vi "Supplementary Fig.9.vi"() -> ()   [LabVIEW 2018]
uses:
  cd616403-dbdb-4a2d-b889-8bc5e4dbac0b.vi
  <vilib>/Analysis/baseanly.llb/Mean (DBL).vi
  <vilib>/Array/Sort 2D Array - Pop Stack.vi
  <vilib>/Array/Sort 2D Array - Push Stack.vi
  <vilib>/Utility/file.llb/Read Delimited Spreadsheet (string).vi
  <vilib>/Utility/file.llb/Write Delimited Spreadsheet (string).vi
  <vilib>/Analysis/NI_AALBase.lvlib
  <vilib>/Analysis/NI_AALPro.lvlib
  <vilib>/gmath/NI_Gmath.lvlib
panel:
  out "appended path":path
  out "coerced(x)":dbl[](array[numeric])=[1.7871616862624315, 4.7491649613370654, 3.3004814514035252, 1.8375936522629628, 3.202316398326516, 4.319522827090855, 3.6552232003410356, 4.668576210850217, 5.083284828825093, 6.10710953942415, 1.646654574018751, 3.7290215132163573, 6.098038325809161, 5.656422627696404, 1.7758128410410414, 3.761570516262, 4.165469016958864, 3.753437357839156, 1.8892827388338778, 4.736459568723037, 1.9574851838284406, 1.920321934057286, 1.925685182031331, 3.788311995806621, 3.0656954505481155, 3.3434841534854978, 3.244966710765227, 1.94311088130418, 3.262816320637847, 1.5462436499858399, 4.548235957251834, 3.6315283681364328, 5.664268399574894, 3.7876699725560314, 1.5612286705468439, 3.287096907045537, 1.6510086873136212, 3.624242770804696, 5.724032802363539, 4.606639647843998, 5.72864322441162, 4.593664726193712, 3.681475732616018, 1.9120549299762257, 6.051355605980825, 4.229281804790069, 3.3406395414558507, 1.8857089065912496, 5.028477399370969, 1.8779605152106047, 1.9111177530654646, 4.664931537320069, 4.186588228645763, 3.2553177687757553, 5.145740103560326, 1.8655992677296291, 1.8046874224504181, 3.0833404640629962, 5.114735680413688, 1.671303972442136, 6.15886900181359, 1.6937395643797195, 3.2536286190286905, 1.842378459360618, 3.7411416491379326, 3.687868246017935, 4.6687925790572375, 1.7586356265470842, 1.8767109641028685, 6.223402134828333, 1.9218572626605044, 3.262014311657234, 1.858320784403082, 4.229963891029505, 1.7347160978595189, 1.685903113936927, 3.700740882251585, 1.7486080037864187, 1.3279294574595724, 3.27544870212411, 3.1368795583033524, 5.616373614885827, 4.268739670631767, 4.253677140988713, 3.6598944224590073, 1.6651274746829139, 4.567994774469708, 1.8542816659595915, 1.688649332258707, 3.29103595985378, 1.8177153438196487, 6.156642024225981, 5.693990388178911, 3.7467283566933944, 1.8453752547517892, 1.917568921369865, 3.2166573059812857, -6.0, 3.89516119392203, 4.232066120234996, 4.139995221043025, 4.973110775936315, 5.608411862084524, 6.134742821848983, 3.291437641822879, 1.8493786914051453, 6.155209143744587, 1.9469302220382134, 3.15342082229652, 1.9749257606375414, 3.343048402338881, 4.2227229180842905, 1.747201555363561, 1.9147522538662338, 1.8587717675188418, 5.662609144117798, 1.9579770221178325, 1.9867431460029874, 3.7904353802213953, 4.230297805342971, 3.2424672304005973, 1.7245832822394196, 5.085249166237611, 1.6080931386501884, 1.613418966188712, 5.140685993693935, -6.0, 1.8719017949112369, 4.2036571121076935, 4.613226980723122, 3.715812337259548, -6.0, 6.061258340225863, 3.7784475546863354, 3.175380674901726, -6.0, 4.615776455361565, 5.184458666423934, 2.025873248470572, 1.73105429451897, 1.716152423032959, 2.036713590493777, 1.574951505953829, 1.8586171256624935, 3.8601284514654104, 4.257991110958849, 1.2065423321612012, 5.611842616698198, 4.579328211355799, 4.111465632573334, 5.146009633606169, 4.567990817904687, 1.9354997588134508, 0.231812761540904, 1.8926221225819462, 3.220052434083975, 3.1463031104018313, 3.22934925835474, 3.327581039341003, 4.345931379092285, 2.0190197998590023, 1.8508399889779195, 1.8366049172096368, 3.1947954331244874, 4.158453183730934, 4.590854029283031, 1.5620256852329995, 1.9893632927815357, 1.659705825153652, 3.795380915100212, 1.195897550086908, 6.0964899066291665, 4.293081716415471, 4.187708236455775, 1.8949490451589543, 5.297148552742282, 3.5382709525514318, 3.578648565876757, 3.277535694974436, 1.707088847431416, 3.7419078216422346, 1.8807526839232078, 6.117955417135745, 3.7912239842840867, 3.6896107042372273, 1.6523256191092637, 1.7960841364158975, 1.636221470769201, 5.155760366117264, 5.656387939814442, 1.3357976408128798, 4.348441122733338, 3.879302402815981, 1.7524323251076086, 3.325504807507367, 1.9436913184974423, 3.773197277176825, 1.6851970426101552, 3.357871833347651, 1.5597183420965208, 3.3109889271775175, 3.7365065137012836, 4.6334044609059575, 1.8003185815047131, 1.7383792054463407, 1.6498374438002832, 3.7494393752685258, 1.460031997854308, 1.7920524290693296, 1.8162541496139923, 0.3871565974248339, 4.612645757412732, 4.6592514227918125, 4.564963074244081, 0.9429870149856682, 1.7270964549130992, 6.048468648027366, 5.04871188235065, 4.240467531757491, 3.270178269411716, 5.0804248855576155, 5.820448008477603, 3.768068761017986, 6.1524394738365356, 4.1177625818053185, 6.111113088204756, 1.5366038643690156, 1.6606280398831155, 3.7487600956387754, 4.757735202780968, 1.945793554112217, 3.807325140809996, 1.8712704526987887, 3.735923451922705, -6.0, 5.115000993235436, 4.380398873391102, 1.953798786138667, 4.636272145582572, 1.8273375076454474, 1.5459102430749714, 6.0846786930998915, 3.0890760065506027, 1.5470917850623196, 3.414232163593886, 1.8784324342398588, 5.568704779949148, 1.7588686726502683, 3.2913100959369586, 3.7322491342602486, 5.661382491336868, 1.4119982524594679, 1.9465745331390063, 1.7300309182128206, 4.696356057813045, 4.964053988335164, 4.695631209986867, 5.6621629936392734, 5.6265410460358325, 4.134527945665677, 4.138785260823419, 4.674190604292248, 1.930554942741988, 5.774946746787386, 4.307050909108307, 3.257989350115037, 1.3904335782414181, 3.6408565707327174, 3.262074232050821, 3.2764631759901555, 1.848577584401121, 1.827328433234382, 1.8960337747362794, 3.3041030370948374, 4.659246088467658, 3.210503304520497, 6.133408069554185, 3.5826212864175275, 6.111857614641569, 1.696478917640413, 3.6241546068461754, 5.22798044456426, 3.7519995544236524, 3.1219975683106997, 5.615946903414847, 3.6701121258372478, 4.697000602278537, 4.753643931101217, 5.656789429450875, 1.808528506417126, 4.7160234241873855, 3.5683886756500516, 5.639204986940518, 4.612624965415669, -6.0, 3.787560696986183, 5.10881077367408, 3.3537508122386126, 1.7718675509127513, 3.729390780351592, 1.1802873430259595, 3.0444549741493296, 4.24672540031586, 5.146264484882083, 3.28179514705405, 4.71404906709892, 5.109900283765078, 3.6140930051711266, 1.946678471551835, 3.6605074662327364, 1.8327673878842443, 3.242524603781917, 5.644941262625613, 1.8207855178820165, 4.7124578651337865, 1.8310254890264943, 1.7233969931626747, 6.084744741056078, 3.7447894548142115, 4.591053763793992, 5.690718937826536, 4.621081782709175, 1.6154774441434179, -6.0, 1.738930340473572, 4.2861274968388114, 4.186865946356676, 5.089454194286781, 1.4444445377463588, 3.2266824238862917, 1.8541422971015722, 6.144774691882833, 6.081983773027188, 5.665405834035932, 3.230297633583582, 1.9813658717460187, 4.268715548550998, 3.1603284853374203, 3.1925795297887505, 4.775281033677114, 4.241797375586176, 4.176880540064573, 1.9201767641917182, 6.085705663824028, 5.7079581669094015, 1.5413908216067886, 5.636004373210665, 5.0663995272902556, 4.76324257120765, 3.788440571838505, 3.220202113342905, 1.4773250647190024, 1.4502453967797377, 1.7988832448499659, 5.6146213167944, 5.075176622438101, 1.6190472574726358, 6.039643381801598, 2.003610467075469, 5.0517553831061734, 0.492511191708194, 6.166115565545919, 3.2517453701832015, 3.2807633335959205, 3.7531912971441037, 1.866488852235544, 1.815261860210051, 1.7154256234981156, 1.8487750622102372, 6.135926272641424, 3.1570698301320657, 1.8960117589378596, 0.3204447869350835, 1.443174883256306, 2.0360349109813636, 5.28182732836023, 5.077250657859839, 0.8087337027630944, 1.8396089759074978, 3.6395594044778523, 1.7408184121349726, 1.793196426632025, 1.893985596206091, 1.7838410092168282, 1.7558360874452674, 3.722918798068077, 4.216885293889205, 5.050524628381662, 5.460371696735989, 5.133147292731508, 3.7043513164181427, 6.087569430540786, 5.162414361098457, 1.930402193876784, 1.8487806604029207, 4.005641262803538, 1.4332832475963648, 3.0590477068872386, 1.8461360713964619, 4.5099930962861565, 1.769126455955212, 5.033360060420678, 1.8190000624294527, 3.255128164822189, 4.212433313348358, -6.0, 3.316188486924122, 3.23019364138835, 3.7957278405824186, 1.4168099822318794, 5.1176017436748795, 4.2556053094661435, 5.093984562350116, 6.052213040115122, 3.1797507208319966, 1.4397455668401162, 1.6665840182464593, 6.153468876985319, 3.7308976534322444, 3.2906244569156007, 3.1549827650297084, 5.5880803202832965, 5.200358521823363, 1.928687791543826, 1.0120576203426224, 3.7468547587589343, 2.014619310619202, 4.664894471832111, 4.154782912356386, 6.116253447268662, 1.7906457672949294, 5.142509396818882, 1.9302839395891997, 4.191792649357379, 6.1438367723348355, 5.107781301970035, 3.6752721725438486, 1.925946883606187, 3.644826317829624, 3.7219899568797676, 3.9084807388586325, 3.2068581232230047, 5.147884754186237, -6.0, -6.0, 5.155258937957506, 4.555483154870481, 4.564905256987634, 1.8124903349442976, 3.154384497999989, 1.7868050385923993, 1.9289894925706583, 4.682905174953122, 6.0099354084690395, 3.3482319844618527, 1.611920203703713, 4.2221213418770445, 4.631661772685009, 1.674581881337848, 3.153515741834732, -6.0, 1.8620458303853011, 5.133997735463562, 1.7070586592824344, 1.8156932061674182, 5.08617481260544, 3.229187606888848, 5.605858992814849, 3.341251367424632, 3.1100966149814386, 5.173982465505348, 1.7834843399537785, 4.176725530975806, -6.0, 1.3606300071078101, 5.614879505481419, 1.8472931155004508, 1.6675136471397716, 3.7647186386378393, 6.123919597813203, 5.612762159529842, 5.690864478125958, 4.226246546698345, 4.255129044053117, 4.224462485105966, 4.694285966418743, 1.7184351611506758, 4.308963598546429, 5.207854509662446, 3.259713201981584, 6.067584503363792, 1.9358964298642602, 4.5663698129989685, 5.559759910512286, 0.3772699976247565, 1.5849254956703018, 1.8099162418539883, 1.9057342223596525, 4.249212707075614, 3.659011694892542, 3.828125478045003, 5.148714404505429, 1.6937199772983755, 6.1305664927082235, 3.753363635354085, 1.8560809944746686, 1.8237788327232272, 1.7476136341099398, 1.9469056547501533, 1.7359181963061763, 3.7685500874730895, 4.612252527392213, 4.169260089075253, 1.6984437289208514, 5.137668501206944, 6.175225181467641, 5.110387621125306, 1.8012932081510782, 1.9170369382742187, 5.173343923381356, 1.6826841787193263, 4.646369542823793, 1.351420947529353, 5.072565356937414, 4.636950999500978, 3.1980169070011675, 1.841894549443889, 5.613278542057316, 1.870856108632458, 1.8811518844658337, 4.642382572974339, 4.574130441897333, 4.6276378076739215, 1.7349303542550565, 5.643352548525211, 3.315670571904706, 1.9605846447982938, 1.7467596358881765, 5.66461413145304, 4.6222431211728585, 4.697659831456345, 1.8597948948572858, 1.2922309214325127, 1.7973128311583562, 5.197177515139583, 5.139577946016122, 5.559318112318645, 1.5024674337519917, 1.7882296419507517, 1.8937981791462262, 4.216665846443737, 4.2049155018749325, 1.2999868932404879, 5.6636902441990875, 3.623030837766795, 3.6766757724641934, 1.5463202033208765, 5.594672564548696, 4.584906066216061, 1.8177443056467912, 1.8551448045518424, 5.642146794473806, 6.15704584106524, 5.650061703435735, 1.1366745358420236, 1.7348907339855077, 3.239356802215263, 1.659981016297658, 1.911891957674333, 5.668550823116212, 5.629572064716126, 5.622544246941823, 6.069322625000074, 3.7102615718886334, 3.1947643045065566, 1.850506717877915, 1.6400817618242793, 5.616024581303818, 1.8316798648455752, 3.318149857639774, 4.26915057172803, 3.693866079422621, 4.179602616586774, 1.7390011604991262, 3.225697530259093, 5.172738614517008, 1.5538744619810934, 3.310744051114857, 3.1686978379815773, 5.129756353458132, 5.70476630271836, 1.7211822468428042, 1.9540532026511654, 3.194357935517832, 3.3174144305947633, 1.9072173522866998, 3.75776587224984, 3.7493526929067933, 5.222013565096699, 4.164303207138102, 5.7397589855477325, 2.0198487241604077, 1.9508862448238076, 1.6488558482717486, 4.27562249979253, 5.669195781941759, 1.9690362793431593, 1.6687988685535902, 4.213065885194019, 1.8584040737295702, 4.654007941777578, 5.691763726913073, 4.736417113100859, 4.676010206847196, 6.071069665582147, 3.7601223339637757, 2.9427278237260164, 1.5312673257734735, 3.2341101643885217, -6.0, 5.707977662889405, 1.9532398118360457, 3.77732645744637, 6.085473348755801, 4.573065587919313, 5.039167075168178, 1.6395538694122245, 5.199620927314441, 1.9150225370062077, 5.662903033924214, 6.086457213036949, 3.3249809624804576, 6.0907846033375215, 3.686328732719376, 1.8096740907194235, 5.598084589983934, 5.153869461545504, 1.9018585596948745, 6.024745716223153, 3.7388530519535834, 1.8746099127797977, 3.069738947349552, 3.758685303480345, 1.7405609825601227, 1.7916819139301732, 2.0682621943565, 1.3596953476098517, 3.801460349644706, 1.8314904420799925, 4.559630609194131, 1.6371015529931428, 4.282149565236064, 3.310959824077987, 4.195632545872944, 3.675388300971693, -6.0, 1.5906428582687027, 5.11076516554976, 3.7338982130897596, 1.739339859535754, 1.9929178807168113, 4.303698457069036, 2.0571649996106194, 4.585681733692552, 3.170164635620533, 1.7444228138520603, 1.9570221804532706, 3.6330383834802196, 3.0712707495155542, 6.104329301798968, 5.110317753811609, 4.282847216418624, 5.670448898132594, 6.149655622163449, 4.593369687158319, 1.510252245324168, 1.7070337893551168, 6.1794066178585645, 1.9956145848613012, 6.0578482755461245, 1.852505501588917, 1.8816482180705145, 6.122879096743778, 1.8346215200335005, 3.2436629994988806, -6.0, 4.192278317351751, 3.2344836319791805, 5.560414501175136, 3.1580028991364926, 1.4085748705902077, 4.2021580092939335, 1.78492288846994, 5.75643114027947, 5.61315456730992, 4.241359051751067, 1.7302088626682521, 1.7218503591678622, 1.883122922564173, 5.643867938880513, 5.210922298309477, 6.072090858700979, 3.3545810131395597, 2.885467323080707, 1.4509108567828515, 1.8736304159176482, 6.076137642531447, 6.137882430759044, 3.2789705623310352, 3.887542932852534, 4.253875746851094, 5.046944625673959, 4.177095937722964, 3.5935793899248356, 1.8016059494695167, 4.250330767438225, 1.437692800983291, 3.72174761890751, 1.9293441848670025, 1.9625802085567017, 1.8721110746230343, 1.9249886744536406, 5.174540869140381, 2.006012042176779, 5.13007539577978, 3.2870833931380727, 1.7818630519774816, 6.205040767643756, 5.105176297628068, 1.6373887593191512, 1.8841608873885956, 0.6705110814541204, 4.662993957636156, 1.4703832768840923, 1.6214092525529635, -6.0, 1.923572672787042, 3.1585131875457373, 3.159249675294813, 3.0540390930783246, 1.1792309783974484, 1.7702569372194743, 3.1351053332356114, 1.9346549306612852, 5.693316291432743, 1.849038947737195, 4.670902458855315, 1.810986802204557, 3.717197118117848, 1.9288065118869488, 3.135066822934636, 1.7198271852013551, 3.766361179281768, 1.7607176128909743, 1.7675972857561029, 1.6868408845616951, 1.784344906730868, 5.59249605929259, 4.641124963216757, 3.686394071664694, 1.8554512138555737, 0.8980543038322548, 3.6350166843770815, 6.102073016901307, 5.670567120812509, 3.6763775562036214, 4.150032234643051, 3.7189935835093366, 3.6866891912543065, 3.4000710703278862, 4.148166318585837, 3.801241472238251, 2.970317740788838, 3.110029085492094, 5.039596460337458, 1.5257935719743616, 6.037572548800155, 3.1167185347135895, 1.8153753225836933, 3.650896403412224, 6.210434884080771, 1.9733572067777208, 6.072734490876358, 5.602695558881499, 0.19812543810824154, 3.5946428480086006, 1.8491402330568831, 4.256581366944582, 6.16299297762625, 3.3177528692463136, 1.8405877309890397, 3.315438376831165, 4.5960155758944, 3.762325605952752, 5.708177595302542, 1.7980308124089122, 4.580172802552053, 4.641906390261374, 5.10610802386794, 1.0689405810335257, 3.756412442700031, 1.6621445716194032, 3.2121212018296186, 1.0905656544893276, 6.109087292438708, 1.7045613830130464, 3.261673161737872, 5.181790291715928, 3.1526217948720956, 1.724238477694529, 5.0516087454053284, 5.60443081840953, 1.891660787597332, 4.628656650854219, 5.167457487372806, 3.7224958534254124, 1.7534798346663736, 3.659894063316376, 5.0922136390437895, 6.143659129937368, 3.7979943254692903, 3.6609603147185115, 1.7469422830568997, 1.7779425434591767, 1.842346443153822, 2.9176004909743227, 6.0771099380718665, 3.8080533872974343, 1.8403395465713333, 1.882529626513101, 1.9907894390633594, 3.1778268390962388, 1.4836044116851346, 3.2347671420248276, 5.047228208512596, -6.0, 3.647858983377213, 1.7092281666032834, 3.277446898096687, 4.764139205803011, 4.220692990286239, 1.937340090770517, 1.8172272616869425, 3.2984281834044937, 1.964154236159909, 1.6877948339082205, 1.721955712903482, 3.147619608788074, 1.8882588676054721, 5.061861465154706, 3.2620324502712643, 1.6535012043312718, 3.7628773180024275, 4.23113043665259, 1.9909072441489264, 1.6480611233110156, 1.568048214922474, 1.9572428199946788, 3.2650535117915815, 1.7491836605066104, 6.064137802913037, -6.0, 3.2375882284288355, 1.5697470552234873, 3.8452072239900326, -6.0, 3.2053157291452625, 5.572436608146442, 1.7583876308208932, 3.2203484445867243, 3.6855622073215066, 1.7137338646345357, 1.8145781931110154, 4.659981336525294, 5.102621410719233, 3.467056992374644, 5.674776916296293, 4.793654377310735, 5.640413965591396, 2.005531196709391, 1.8554325788835098, 3.242106531535169, 1.8098521622977441, 5.6989554698277765, 4.664518804707001, 3.2844750262388596, 5.628831986318144, 5.562795248124345, 6.065481335243661, 3.6801115696274476, 5.20422170449058, 3.856715864977252, 5.643818261701583, 1.847629847764977, 5.112968981436306, 6.08465903943604, 1.8369373419325807, 4.668592928087283, 1.8880375974637427, 3.0531999232556237, 3.6489968506814687, 1.7570638791239357, 1.8487613063445654, 1.8504654967727336, 5.642404851857281, 3.787394442355481, 0.7338503027874327, 3.6946134241299573, 4.175183268067918, 1.853993158131384, 4.728520025961949, 1.7998641995834261, 3.064062965934454, 4.8242654572654855, 1.840000263076598]
  in  "6peak boundary PE":dbl[](array[numeric])=[3.3500000000000036, 3.9500000000000024, 4.400000000000004, 5.0, 5.350000000000005, 7.0000000000000036] format="%_3g"
  in  "8peak boundary PE":dbl[](array[numeric])=[2.1999999999999997, 3.0999999999999996, 3.5999999999999996, 4.100000000000001, 4.450000000000001, 5.000000000000002, 5.350000000000002, 7.0] format="%_3g"
  in  "filename appendix":string
  in  "6peak(T)/8peak(F)":bool
  in  "8peak boundary FL":dbl[](array[numeric])=[2.8000000000000003, 3.5, 4.0, 4.4, 4.85, 5.35, 5.8500000000000005, 7.0] format="%_3g"
  in  "8peak-PE":dbl[](array[numeric])=[487.0, 1474.0, 4516.0, 11260.0, 34341.0, 107608.0, 260461.0]
  in  "8peak-FL":dbl[](array[numeric])=[771.0, 2106.0, 6262.0, 15183.0, 45292.0, 136258.0, 291042.0]
  in  "frame":i32=13
  in  "all":bool
  in  "channel":i32
  in  "file path":path
  in  "length(y) for bg calc":i32=24
  in  "length(x) for bg calc":i32=30
  out "loop index for stat analysis":i32=66
  out "loop index":i32=2999
  in  "load file":bool
  in  "save extracted data":bool
  out "size(s)":i32[](array[numeric])=[915, 7]
  in  "gating":bool=TRUE
  in  "index":i32=2
  in  "gating":T1(array[cluster])=[{"limit"=FALSE, "low"=0.0, "up"=500.0, "feature"=0}, {"limit"=TRUE, "low"=0.0, "up"=180.0, "feature"=1}, {"limit"=FALSE, "low"=0.0, "up"=1000000000.0, "feature"=2}, {"limit"=FALSE, "low"=0.30000000000000016, "up"=2.0, "feature"=3}, {"limit"=FALSE, "low"=0.0, "up"=1000000000.0, "feature"=4}, {"limit"=FALSE, "low"=27.0, "up"=60.0, "feature"=5}, {"limit"=FALSE, "low"=20.0, "up"=60.0, "feature"=6}] {"feature" items=["flow position", "seg area", "encircled intensity", "ratio", "total intensity", "peak x pos", "peak y pos"]}
  in  "feature names":string[](array[string])=["flow position", "seg area", "encircled intensity", "ratio", "total intensity", "peak x pos", "peak y pos"]
  in  "aperture diameter":dbl=10.0
  in  "Threshold Limits":cluster{"Lower value":sgl, "Upper value":sgl}={"Lower value"=0.29999992, "Upper value"=65000.0} {"Upper value" format="%.2f"; "Lower value" format="%.2f"}
  in  "in1":T2={"Niblack Dev Fac"=0.5, "Window"={"Width"=20, "Height"=20}, "Sauvola Dev Rng"=6000.0, "adaptive"=FALSE, "Method (Niblack)"=0} {"Method (Niblack)" items=["Niblack", "Background Correction", "Sauvola"]}
  in  "post proc1":T3={"trunc for ch2 masking"=[0, 0, 0, 0], "Erosion(pre)"=2, "Op"=enum."Erode", "post proc"=FALSE, "move x/y"=[0, 0], "conv"=FALSE, "Conn"=TRUE, "iteration"=1, "Erosion(post)"=0}
  in  "seg meth":T4={"norm for thresh"=TRUE, "use thresh formula"=FALSE, "thresh"=0.2500000000000001, "man thresh"=TRUE, "Meth"=0, "upper lim"=67100} {"Meth" items=["clustering", "entropy", "metric", "moments", "inter-class variance"]; "thresh" format="%_3g"}
  in  "lpf 1":cluster{"cut":dbl, "lpf":bool, "odr":i32}={"cut"=0.25000010000000006, "lpf"=FALSE, "odr"=2} {"cut" min=1e-07 max=0.4999 step=0.01 format="%_2g"}
  in  "shift":i32[](array[numeric])=[5, 5]
  in  "image lpf":cluster{"cut":dbl, "lpf":bool, "odr":i32}={"cut"=0.050000100000000006, "lpf"=TRUE, "odr"=2} {"cut" min=1e-07 max=0.4999 step=0.01 format="%_3g"}
  in  "6peak-PE":dbl[](array[numeric])=[3236.0, 10754.0, 34842.0, 104483.0, 245894.0]
  in  "num of frames to be processed":u32=3000
  in  "upper limit 3":sgl=12000.0
  in  "lower limit 3":sgl
  out "R^2":dbl=0.9853992563567322
  out "peak positions":dbl[](array[numeric])=[2.953516131979112, 3.2640324566935828, 3.7340171554472747, 4.2247958019394325, 4.65775156331877, 5.12226558332707, 5.854659621300674]
  out "MESF":dbl=65.28474142641139
  in  "bkank position":dbl=1.8700000000000017 format="%_3g"
  in  "6peak boundary FL":dbl[](array[numeric])=[3.3500000000000036, 3.9500000000000024, 4.400000000000004, 5.0, 5.350000000000005, 7.0000000000000036] format="%_3g"
  in  "6peak-FL":dbl[](array[numeric])=[4447.0, 14227.0, 46322.0, 133924.0, 276897.0]
  in  "offset":dbl format="%#_13g"
  out "Histogram":T5(graph)={"X Values"=array[600 elements], "Histogram: h(x)"=[19, 0, 0, 0, 0, 0, 0, 0, 0, 0, 0, 0, 0, 0, 0, 0, 0, 0, 0, 0, 0, 0, 0, 0, 0, 0, 0, 0, 0, 0, 0, 0, 0, 0, 0, 0, 0, 0, 0, 0, 0, 0, 0, 0, 0, 0, 0, 0, 0, 0, 0, 0, 0, 0, 0, 0, 0, 0, 0, 0, 0, 0, 0, 0, 0, 0, 0, 0, 0, 0, 0, 0, 0, 0, 0, 0, 0, 0, 0, 0, 0, 0, 0, 0, 0, 0, 0, 0, 0, 0, 0, 0, 0, 0, 0, 0, 0, 0, 0, 0, 0, 0, 0, 0, 0, 0, 0, 0, 0, 0, 0, 0, 0, 0, 0, 0, 0, 0, 0, 0, 0, 0, 0, 0, 0, 0, 0, 0, 0, 0, 0, 0, 0, 0, 0, 0, 0, 0, 0, 0, 0, 0, 0, 0, 0, 0, 0, 0, 0, 0, 0, 0, 0, 0, 0, 0, 0, 0, 0, 0, 0, 0, 0, 0, 0, 0, 0, 0, 0, 0, 0, 0, 0, 0, 0, 0, 0, 0, 0, 0, 0, 0, 0, 0, 0, 0, 0, 0, 0, 0, 0, 0, 0, 0, 0, 0, 0, 0, 0, 0, 0, 0, 0, 0, 0, 0, 0, 0, 0, 0, 0, 0, 0, 0, 0, 0, 0, 0, 0, 0, 0, 0, 0, 0, 0, 0, 0, 0, 0, 0, 0, 0, 0, 0, 0, 0, 0, 0, 0, 0, 0, 0, 0, 0, 0, 0, 0, 0, 0, 0, 0, 0, 0, 0, 0, 0, 0, 0, 0, 0, 0, 0, 0, 0, 0, 0, 0, 0, 0, 0, 0, 0, 0, 0, 0, 0, 0, 0, 0, 0, 0, 0, 0, 0, 0, 0, 0, 0, 0, 0, 0, 0, 0, 0, 0, 0, 0, 0, 0, 0, 0, 0, 0, 0, 1, 1, 0, 0, 0, 0, 1, 0, 0, 2, 0, 0, 0, 0, 1, 0, 0, 0, 0, 0, 0, 0, 0, 1, 0, 0, 1, 0, 0, 0, 1, 0, 0, 0, 1, 0, 1, 0, 0, 0, 1, 0, 1, 0, 1, 0, 1, 0, 2, 2, 0, 0, 0, 1, 1, 1, 2, 2, 1, 2, 2, 6, 2, 2, 2, 3, 6, 6, 2, 5, 5, 10, 8, 10, 10, 20, 15, 7, 19, 17, 18, 28, 16, 13, 13, 16, 16, 4, 9, 4, 2, 1, 1, 0, 0, 0, 0, 0, 0, 0, 0, 0, 0, 0, 0, 0, 0, 0, 0, 0, 0, 0, 0, 0, 0, 0, 0, 0, 0, 0, 0, 0, 0, 0, 0, 0, 0, 0, 0, 0, 0, 0, 1, 1, 1, 0, 1, 0, 0, 1, 4, 4, 1, 4, 4, 11, 5, 8, 8, 14, 12, 11, 7, 12, 5, 3, 0, 1, 1, 0, 1, 0, 0, 0, 1, 1, 4, 1, 6, 7, 10, 10, 5, 12, 15, 12, 10, 4, 1, 3, 1, 2, 1, 0, 0, 0, 0, 1, 0, 0, 0, 0, 2, 3, 6, 6, 9, 9, 9, 8, 7, 3, 2, 2, 0, 1, 0, 0, 0, 0, 0, 1, 0, 1, 8, 8, 7, 7, 7, 12, 3, 6, 2, 4, 4, 1, 0, 1, 0, 0, 0, 0, 0, 0, 2, 0, 0, 4, 7, 5, 7, 12, 8, 9, 6, 5, 3, 1, 0, 1, 1, 0, 0, 0, 0, 0, 0, 0, 1, 0, 0, 0, 0, 5, 2, 8, 12, 10, 15, 5, 6, 2, 1, 2, 0, 0, 1, 0, 0, 0, 0, 0, 0, 0, 0, 1, 3, 4, 10, 11, 8, 7, 10, 4, 0, 3]}
  in  "intervals":i32=600
  out "image":dbl[][](graph)
  in  "stop":bool
  out "pix num (y)":u32=88
  out "pix num(x)":u32=100
  out "# of frames":u32=3000
  out "#of chnnels":u32=2
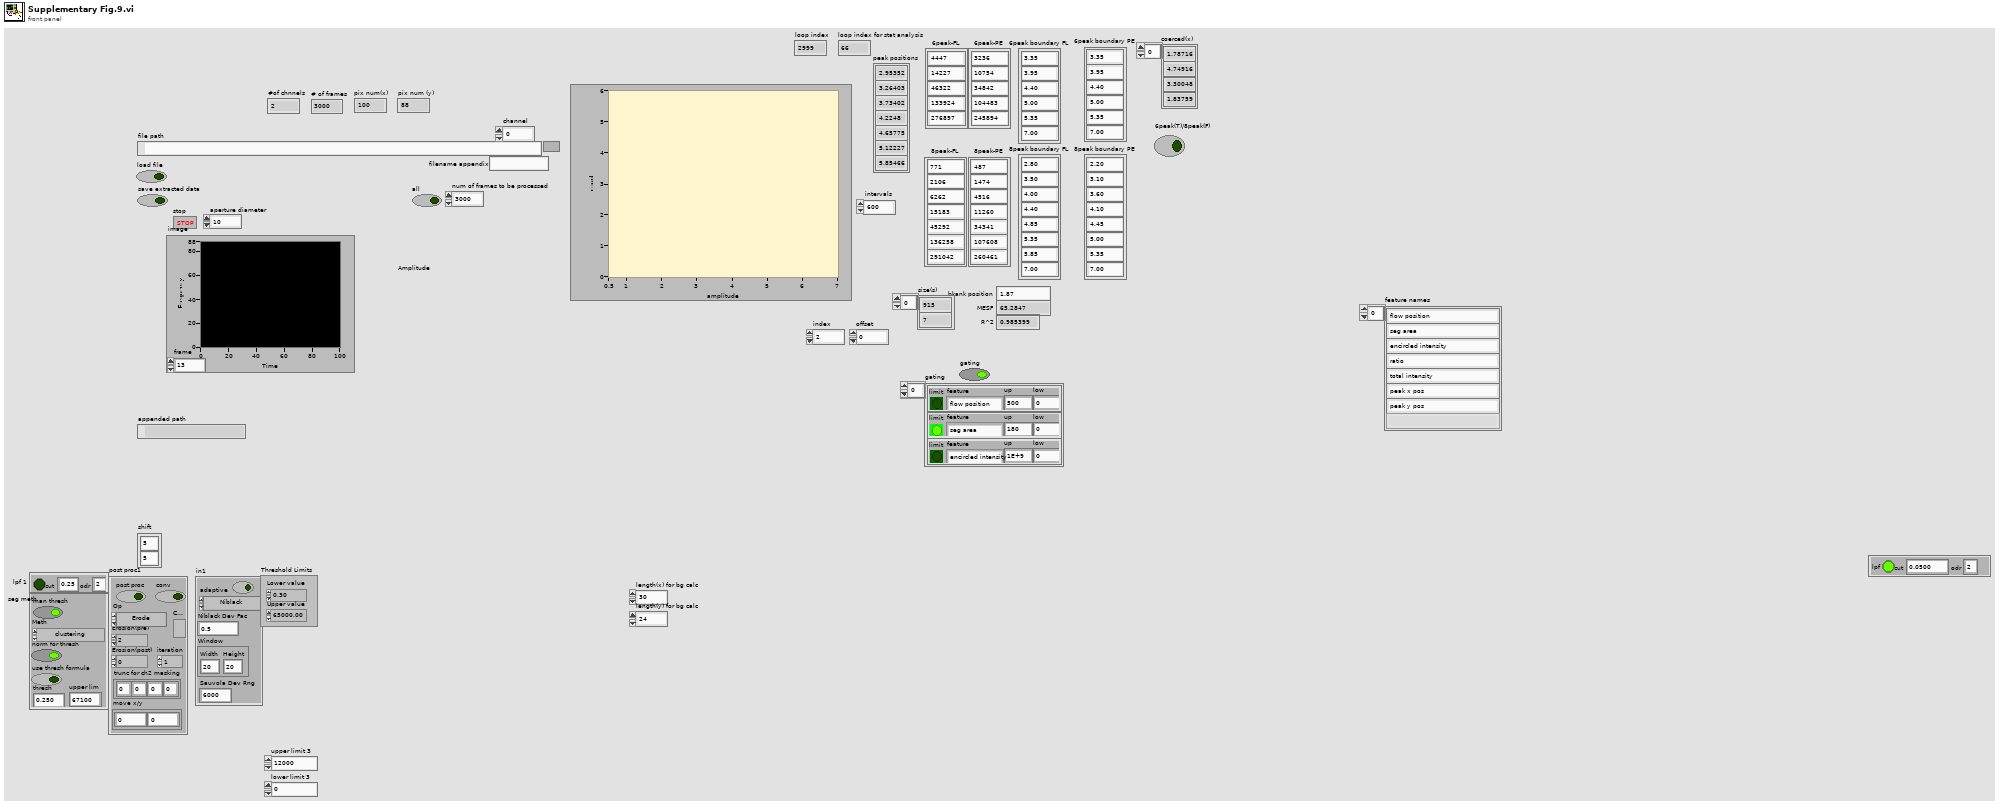
[diagram p1: front panel]
types:
  T1 = cluster{"limit":bool, "low":dbl, "up":dbl, "feature":i32}[]
  T2 = cluster{"Niblack Dev Fac":dbl, "Window":cluster{"Width":i32, "Height":i32}, "Sauvola Dev Rng":dbl, "adaptive":bool, "Method (Niblack)":u32}
  T3 = cluster{"trunc for ch2 masking":i32[], "Erosion(pre)":i32, "Op":enum32{"AutoM", "Close", "Dilate", "Erode", "Gradient", "Gradient out", "Gradient in", "Hit miss", "Open", "PClose", "POpen", "Thick", "Thin"}, "post proc":bool, "move x/y":i32[], "conv":bool, "Conn":bool, "iteration":i32, "Erosion(post)":i32}
  T4 = cluster{"norm for thresh":bool, "use thresh formula":bool, "thresh":dbl, "man thresh":bool, "Meth":i32, "upper lim":i32}
  T5 = cluster{"X Values":dbl[], "Histogram: h(x)":i32[]}
  T6 = enum16{"big-endian, network order", "native, host order", "little-endian"}
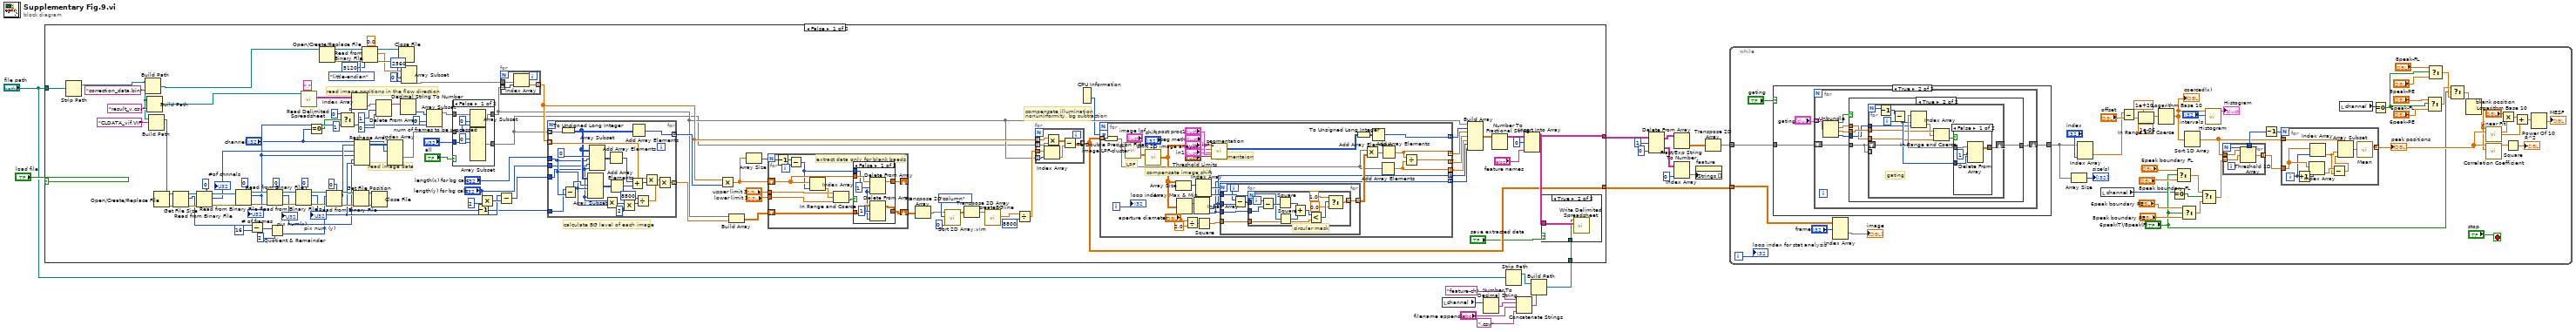
[diagram p0: block diagram]
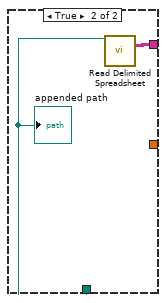
[diagram p5: hidden frame]
diagram:
  n1 = local read "channel"() -> (w6:i32)
  n2 = Number To Decimal String(number=w6) -> (decimal integer string=w5:string)  [unwired: 1 in]
  n3 = Strip Path(path="file path") -> (stripped path=w1:path)  [unwired: 1 out]
  n4 = Concatenate Strings("feature-ch" ("name or relative path"), w5, "filename appendix", ".csv" ("name or relative path")) -> (w7:string)
  n5 = Build Path(base path=w1, name or relative path=w7) -> (appended path=w9:path)
  n6 = case shown="False" "load file" {
    tunnel: [w56 w243] -> w20
    tunnel: [w55 _] -> w19
    tunnel: w9 -> [w50 w242]
    tunnel: "file path" -> [w22 _]
    frame False {
      # "compensate illumination nonunirformity, bg subtraction"
      # "calculate BG level of each image"
      # "read image data"
      # "read image positions in the flow direction"
      n7 = Strip Path(path=w22) -> (stripped path=w27:path)  [unwired: 1 out]
      n8 = Build Path(base path=w27, name or relative path="correction_data.bin") -> (appended path=w93:path)
      n9 = Build Path(base path=w27, name or relative path="result_v.csv") -> (appended path=w100:path)
      n10 = Build Path(base path=w27, name or relative path="CLDATA_vif.VIF") -> (appended path=w128:path)
      n11 = Open/Create/Replace File(file path (use dialog)=w128) -> (refnum out=w111:refnum<file>, error out=w110:errorcluster)  [unwired: 5 in, 1 out]
      n12 = Get File Size(file=w111, error in=w110) -> (refnum out=w109:refnum<file>, size (in bytes)=w107:i64, 0:w108:errorcluster)
      n13 = Read from Binary File(5:u32 0, 8:w108, 11:w109) -> (0:w119:errorcluster, 2:w101:u32, 3:w118:refnum<file>)  [unwired: 3 in, 1 out]
      "#of chnnels" <- w101
      n14 = Read from Binary File(5:u32 0, 8:w119, 11:w118) -> (0:w120:errorcluster, 2:w36:u32, 3:w122:refnum<file>)  [unwired: 3 in, 1 out]
      "# of frames" <- w36
      n15 = Subtract(x=w107, y=i64 16) -> (x-y=w105:i64)
      n16 = Read from Binary File(5:u32 0, 8:w120, 11:w122) -> (0:w123:errorcluster, 2:w41:u32, 3:w121:refnum<file>)  [unwired: 3 in, 1 out]
      "pix num(x)" <- w41
      n17 = Quotient & Remainder(x=w105, y=i64 2) -> (floor(x/y)=w37:i64)  [unwired: 1 out]
      n18 = Read from Binary File(5:u32 0, 8:w123, 11:w121) -> (0:w116:errorcluster, 2:w44:u32, 3:w117:refnum<file>)  [unwired: 3 in, 1 out]
      "pix num (y)" <- w44
      n19 = call-poly <vilib>:"Read Delimited Spreadsheet.vi"("file path (dialog if empty)"=w100, "delimiter (\\t)"="," ("delimiter (\\t)")) -> ("all rows"=w98:string[][])  [unwired: 8 in, 5 out]
      n20 = Equal To 0?(x="channel") -> (x = 0?=w23:bool)
      n21 = Open/Create/Replace File(file path (use dialog)=w93) -> (refnum out=w84:refnum<file>, error out=w83:errorcluster)  [unwired: 5 in, 1 out]
      n22 = Read from Binary File(5:u16 0, 8:w116, 10:w37, 11:w117) -> (0:w114:errorcluster, 2:w102:u16[], 3:w115:refnum<file>)  [unwired: 2 in, 1 out]
      n23 = Select(t=0 ("disabled index (col)"), s=w23, f=1 ("disabled index (col)")) -> (s? t:f=w21:i32)
      n24 = Index Array(array=w98, index (col)=w21) -> (element=w97:string[])  [unwired: 1 in]
      n25 = Get File Position(4:w114, 7:w115) -> (0:w112:errorcluster, 3:w113:refnum<file>)  [unwired: 1 out]
      n26 = Reshape Array(w102, w101, w36, w41, w44) -> (w38:u16[][][][])
      n27 = Read from Binary File(5:sgl 0.0, 8:w83, 9:T6."little-endian" ("byte order (0:big-endian, network order)"), 10:5120 ("count (1)"), 11:w84) -> (0:w90:errorcluster, 2:w87:sgl[], 3:w91:refnum<file>)  [unwired: 1 in, 1 out]
      n28 = Close File(refnum=w113, error in=w112) -> ()  [unwired: 2 out]
      n29 = Delete From Array(array=w97, length=1, index=0) -> (array with subset deleted=w94:string[])  [unwired: 1 out]
      n30 = Index Array(array=w38, index (dim 0)="channel") -> (element=w54:u16[][][])  [unwired: 3 in]
      n31 = Close File(refnum=w91, error in=w90) -> ()  [unwired: 2 out]
      n32 = Decimal String To Number(string=w94) -> (number=w78:i32[])  [unwired: 2 in, 1 out]
      n33 = Array Subset(array=w87, index=0, length=2560) -> (w82:sgl[])
      n34 = Array Subset(array=w78, index=0, length=w36) -> (w52:i32[])
      n35 = case shown="False" "all" {
        tunnel: w54 -> [w135 w136]
        tunnel: w52 -> [w134 w137]
        tunnel: [w133 w137] -> w34
        tunnel: [w132 w136] -> w32
        tunnel: "num of frames to be processed" -> [w131 _]
        frame False {
          n36 = Array Subset(array=w134, index=0, length=w131) -> (w133:i32[])
          n37 = Array Subset(array=w135, index (dim 0)=0 ("index"), length (dim 0)=w131) -> (w132:u16[][][])  [unwired: 4 in]
        }
        frame True {
        }
      }
      n38 = Decrement(x=w41) -> (x-1=w40:u32)
      n39 = Multiply(x="length(y) for bg calc", y=2) -> (x*y=w45:i32)
      n40 = Subtract(x=w44, y=w45) -> (x-y=w43:u32)
      n41 = for {
        tunnel: w34 -> [w218] mode=indexing
        tunnel: w82 -> [w219]
        tunnel: [w217] -> w77 mode=indexing
        n42 = Index Array(array=w219, index=w218) -> (element=w217:sgl)
      }
      n43 = for {
        tunnel: w32 -> [w241] mode=indexing
        tunnel: [w234] -> w67 mode=indexing
        tunnel: w77 -> [w232] mode=indexing
        tunnel: [w230] -> w74 mode=indexing
        tunnel: "length(x) for bg calc" -> [w223]
        tunnel: "length(y) for bg calc" -> [w222]
        tunnel: w43 -> [w221]
        tunnel: w40 -> [w220]
        n44 = To Unsigned Long Integer(number=w241) -> (unsigned 32bit integer=w231:u32[][])
        n45 = Subtract(x=w220, y=w223) -> (x-y=w224:u32)
        n46 = Array Subset(array=w231, index (row)=w224, length (row)=w223, length (col)=w221) -> (w237:u32[][])  [unwired: 1 in]
        n47 = Array Subset(array=w231, index (row)=0 ("index"), length (row)=w223, index (col)=w222, length (col)=w221) -> (w239:u32[][])
        n48 = Multiply(x=w221, y=w223) -> (x*y=w229:u32)
        n49 = Add Array Elements(numeric array=w239) -> (sum=w238:u32)
        n50 = Add Array Elements(numeric array=w237) -> (sum=w235:u32)
        n51 = Multiply(x=w229, y=2) -> (x*y=w227:u32)
        n52 = Add(x=w238, y=w235) -> (x+y=w236:u32)
        n53 = Add Array Elements(numeric array=w231) -> (sum=w230:u32)
        n54 = Divide(x=8800, y=w227) -> (x/y=w225:dbl)
        n55 = Multiply(x=w232, y=w236) -> (x*y=w233:sgl)
        n56 = Multiply(x=w233, y=w225) -> (x*y=w234:dbl)
      }
      n57 = Multiply(x=w77, y=w74) -> (x*y=w53:sgl[])
      n58 = Build Array(w34, w67) -> (w39:dbl[][])
      n59 = Array Size(array=w53) -> (size(s)=w70:i32)
      n60 = for {
        N: w70 -> [w191]
        shift-right: [w192] -> _
        shift-left: w53 -> [w196]
        shift-right: [w193] -> w48
        shift-left: w39 -> [w194]
        tunnel: "lower limit 3" -> [w190]
        tunnel: "upper limit 3" -> [w189]
        i -> [w199]
        # "extract data only for blank baeds"
        n61 = Decrement(x=w191) -> (x-1=w200:i32)
        n62 = Subtract(x=w200, y=w199) -> (x-y=w195:i32)
        n63 = Index Array(array=w196, index=w195) -> (element=w198:sgl)
        n64 = In Range and Coerce(upper limit=w189, x=w198, lower limit=w190) -> (In Range?=w197:bool)  [unwired: 1 out]
        n65 = case shown="False" w197 {
          tunnel: w196 -> [w207 w209]
          tunnel: w195 -> [w201 _]
          tunnel: w194 -> [w205 w208]
          tunnel: [w203 w208] -> w193
          tunnel: [w202 w209] -> w192
          frame False {
            n66 = Delete From Array(array=w205, length=1, index (col)=w201) -> (array with subset deleted=w203:dbl[][])  [unwired: 1 in, 1 out]
            n67 = Delete From Array(array=w207, length=1, index=w201) -> (array with subset deleted=w202:sgl[])  [unwired: 1 out]
          }
          frame True {
          }
        }
      }
      n68 = Transpose 2D Array(2D array=w48) -> (transposed array=w49:dbl[][])
      n69 = call "Sort 2D Array.vim"("index"=0, "dimension to index (column)"=enum16{"column", "row"}."column", "2D array"=w49) -> ("sorted 2D array"=w79:dbl[][])  [unwired: 7 in, 1 out]
      n70 = Transpose 2D Array(2D array=w79) -> (transposed array=w73:dbl[][])
      n71 = call "createBGline.vi"("all rows"=w73) -> ("Array"=w71:dbl[])  [unwired: 8 in, 2 out]
      n72 = Divide(x=w71, y=8800) -> (x/y=w76:dbl[])
      n73 = for {
        tunnel: w32 -> [w216] mode=indexing
        tunnel: w77 -> [w215] mode=indexing
        tunnel: w76 -> [w212]
        tunnel: w34 -> [w211] mode=indexing
        tunnel: [w210] -> w55 mode=indexing
        n74 = Index Array(array=w212, index=w211) -> (element=w213:dbl)
        n75 = Multiply(x=w215, y=w216) -> (x*y=w214:sgl[][])
        n76 = Subtract(x=w214, y=w213) -> (x-y=w210:dbl[][])
      }
      n77 = CPU Information() -> (6:w31:i32)  [unwired: 3 out]
      n78 = for {
        tunnel: w55 -> [w147] mode=indexing
        tunnel: [w146] -> w66 mode=indexing
        tunnel: [w145] -> w64 mode=indexing
        tunnel: [w144] -> w65 mode=indexing
        tunnel: [w143] -> w63 mode=indexing
        tunnel: [w142] -> w62 mode=indexing
        tunnel: [w141] -> w61 mode=indexing
        workers-P: w31 -> [_]
        i -> [w140]
        # "segmentaion"
        # "compensate image shift"
        # "LPF"
        n79 = To Double Precision Float(number=w147) -> (double precision float=w148:dbl[][])
        n80 = call "image LPF-cluster.vi"("image lpf"="image lpf", "input"=w148) -> ("output"=w168:dbl[][])  [unwired: 1 in]
        n81 = call "shift 2D image arrayin.vi"("Array in"=w168, "shift"="shift") -> ("Array out"=w155:dbl[][])
        n82 = Array Size(array=w155) -> (size(s)=w158:i32[])
        n83 = Array Max & Min(array=w155) -> (max index (indices)=w152:i32[])  [unwired: 3 out]
        n84 = Divide(x="aperture diameter", y=2.0) -> (x/y=w161:dbl)
        n85 = Index Array(array=w152) -> (element #1=w142:i32, element #2=w141:i32)  [unwired: 2 in]
        n86 = Index Array(array=w158) -> (element #1=w157:i32, element #2=w156:i32)  [unwired: 2 in]
        n87 = Square(x=w161) -> (x^2=w162:dbl)
        n88 = call "segmentation.vi"("unmixed ch2"=w155, "segmentation method"="seg meth", "image lpf"="lpf 1", "post processing"="post proc1", "input cluster"="in1", "Threshold Limits"="Threshold Limits") -> ("Array"=w150:u8[][])  [unwired: 7 in, 2 out]
        n89 = for {
          N: w157 -> [_]
          tunnel: w142 -> [w176]
          tunnel: [w174] -> w153 mode=indexing
          tunnel: w162 -> [w173]
          tunnel: w156 -> [w172]
          tunnel: w141 -> [w170]
          i -> [w171]
          # "circular mask"
          n90 = Subtract(x=w171, y=w176) -> (x-y=w175:i32)
          n91 = for {
            N: w172 -> [_]
            tunnel: w175 -> [w180]
            tunnel: [w182] -> w174 mode=indexing
            tunnel: w173 -> [w185]
            tunnel: w170 -> [w179]
            i -> [w178]
            n92 = Subtract(x=w178, y=w179) -> (x-y=w181:i32)
            n93 = Square(x=w181) -> (x^2=w188:i32)
            n94 = Square(x=w180) -> (x^2=w187:i32)
            n95 = Add(x=w188, y=w187) -> (x+y=w186:i32)
            n96 = Less?(x=w186, y=w185) -> (x < y?=w184:bool)
            n97 = Select(t=1.0 ("f"), s=w184, f=0.0) -> (s? t:f=w182:dbl)
          }
        }
        n98 = To Unsigned Long Integer(number=w150) -> (unsigned 32bit integer=w149:u32[][])
        n99 = Multiply(x=w148, y=w153) -> (x*y=w151:dbl[][])
        n100 = Add Array Elements(numeric array=w149) -> (sum=w146:u32)
        n101 = Add Array Elements(numeric array=w148) -> (sum=w143:dbl)
        n102 = Add Array Elements(numeric array=w151) -> (sum=w144:dbl)
        n103 = Divide(x=w144, y=w143) -> (x/y=w145:dbl)
        "loop index" <- w140
      }
      n104 = Build Array(w34, w66, w65, w64, w63, w62, w61) -> (w58:dbl[][])
      n105 = Number To Fractional String(number=w58) -> (F-format string=w59:string[][])  [unwired: 3 in]
      n106 = Insert Into Array(array=w59, index (col)=0 ("index (row)"), new element="feature names") -> (w56:string[][])  [unwired: 1 in]
      n107 = case shown="True" "save extracted data" {
        tunnel: w56 -> [_ w139]
        tunnel: w50 -> [_ w138]
        frame False {
        }
        frame True {
          n108 = call-poly <vilib>:"Write Delimited Spreadsheet.vi"("file path (dialog if empty)"=w138, "2D data"=w139) -> ()  [unwired: 12 in, 2 out]
        }
      }
    }
    frame True {
      n109 = call-poly <vilib>:"Read Delimited Spreadsheet.vi"("file path (dialog if empty)"=w242) -> ("all rows"=w243:string[][])  [unwired: 9 in, 5 out]
      "appended path" <- w242
    }
  }
  n110 = Delete From Array(array=w20, length=1, index (col)=0 ("disabled index (col)")) -> (deleted portion=w15:string[][], array with subset deleted=w16:string[][])  [unwired: 1 in]
  n111 = Fract/Exp String To Number(string=w16) -> (number=w13:dbl[][])  [unwired: 3 in, 1 out]
  n112 = Index Array(array=w15, index (col)=0 ("disabled index (col)")) -> (element=w11:string[])  [unwired: 1 in]
  n113 = property on="feature" class="Ring (strict)"("Strings []"=w11) -> ()  [unwired: 2 in, 2 out]
  n114 = Transpose 2D Array(2D array=w13) -> (transposed array=w12:dbl[][])
  n115 = while {
    tunnel: w19 -> [w271]
    tunnel: w12 -> [w266]
    i -> [w264]
    stop <- "stop" stop-if-true
    n116 = case shown="True" "gating" {
      tunnel: [w296 w299] -> w265
      tunnel: w266 -> [w296 w298]
      frame False {
      }
      frame True {
        n117 = for {
          shift-right: [w305] -> w299
          shift-left: w298 -> [w306]
          tunnel: "gating" -> [w304] mode=indexing
          n118 = Unbundle(w304) -> ("limit"=w303:bool, "low"=w302:dbl, "up"=w301:dbl, "feature"=w300:i32)
          n119 = case shown="True" w303 {
            tunnel: [w307 w311] -> w305
            tunnel: w306 -> [w307 w312]
            tunnel: w301 -> [_ w310]
            tunnel: w302 -> [_ w309]
            tunnel: w300 -> [_ w308]
            frame False {
            }
            frame True {
              n120 = for {
                N -> [w323]
                shift-right: [w319] -> w311
                shift-left: w312 -> [w321]
                tunnel: w312 -> [_] mode=indexing
                tunnel: w310 -> [w317]
                tunnel: w309 -> [w315]
                tunnel: w308 -> [w313]
                i -> [w322]
                # "gating"
                n121 = Decrement(x=w323) -> (x-1=w318:i32)
                n122 = Subtract(x=w318, y=w322) -> (x-y=w320:i32)
                n123 = Index Array(array=w321, index (row)=w320, index (col)=w313) -> (element=w316:dbl)
                n124 = In Range and Coerce(upper limit=w317, x=w316, lower limit=w315) -> (In Range?=w314:bool)  [unwired: 1 out]
                n125 = case shown="False" w314 {
                  tunnel: w321 -> [w327 w328]
                  tunnel: w320 -> [w325 _]
                  tunnel: [w326 w328] -> w319
                  frame False {
                    n126 = Delete From Array(array=w327, length=1, index (row)=w325) -> (array with subset deleted=w326:dbl[][])  [unwired: 1 in, 1 out]
                  }
                  frame True {
                  }
                }
              }
            }
          }
        }
      }
    }
    n127 = Index Array(array=w271, index (dim 0)="frame") -> (element=→"image":dbl[][])  [unwired: 2 in]
    n128 = Array Size(array=w265) -> (size(s)=→"size(s)":i32[])
    n129 = Index Array(array=w265, index (col)="index") -> (element=w272:dbl[])  [unwired: 1 in]
    n130 = local read "channel"() -> (w247:i32)
    n131 = Subtract(x=w272, y="offset") -> (x-y=w291:dbl[])
    n132 = In Range and Coerce(upper limit=1e+20, x=w291, lower limit=1e-06) -> (coerced(x)=w277:dbl[])  [unwired: 1 out]
    n133 = Logarithm Base 10(1:w277) -> (0:w244:dbl[])
    "coerced(x)" <- w244
    n134 = Equal To 0?(x=w247) -> (x = 0?=w246:bool)
    n135 = Select(t="6peak boundary FL", s="6peak(T)/8peak(F)", f="8peak boundary FL") -> (s? t:f=w249:dbl[])
    n136 = Select(t="6peak boundary PE", s="6peak(T)/8peak(F)", f="8peak boundary PE") -> (s? t:f=w248:dbl[])
    n137 = Sort 1D Array(array=w244) -> (sorted array=w286:dbl[])
    n138 = Select(t=w249, s=w246, f=w248) -> (s? t:f=w245:dbl[])
    n139 = call <vilib>:"Histogram.vi"("intervals"="intervals", "X"=w244) -> ("Histogram Graph"=→"Histogram":T5)  [unwired: 6 in, 3 out]
    n140 = for {
      N -> [w338]
      tunnel: w286 -> [w341]
      tunnel: w245 -> [w340] mode=indexing
      tunnel: [w339] -> w287 mode=indexing
      tunnel: [w338] -> w288
      n141 = Threshold 1D Array(2:w340, 3:w341) -> (0:w339:dbl)  [unwired: 1 in]
    }
    n142 = Decrement(x=w288) -> (x-1=w289:i32)
    n143 = for {
      N: w289 -> [_]
      tunnel: w287 -> [w334]
      tunnel: w286 -> [w337]
      tunnel: [w335] -> w285 mode=indexing
      i -> [w332]
      n144 = Increment(x=w332) -> (x+1=w333:i32)
      n145 = Index Array(array=w334, index=w333) -> (element=w331:dbl)
      n146 = Index Array(array=w334, index=w332) -> (element=w329:dbl)
      n147 = Subtract(x=w331, y=w329) -> (x-y=w330:dbl)
      n148 = Array Subset(array=w337, index=w329, length=w330) -> (w336:dbl[])
      n149 = call-poly <vilib>:"Mean.vi"("X"=w336) -> ("mean"=w335:dbl)  [unwired: 1 out]
    }
    "peak positions" <- w285
    n150 = local read "channel"() -> (w263:i32)
    n151 = Equal To 0?(x=w263) -> (x = 0?=w256:bool)
    n152 = Select(t="6peak-FL", s=w256, f="6peak-PE") -> (s? t:f=w254:dbl[])
    n153 = Select(t="8peak-FL", s=w256, f="8peak-PE") -> (s? t:f=w255:dbl[])
    n154 = Select(t=w254, s="6peak(T)/8peak(F)", f=w255) -> (s? t:f=w253:dbl[])
    n155 = Logarithm Base 10(1:w253) -> (0:w280:dbl[])
    n156 = call <vilib>:"Linear Fit.vi"("Y"=w280, "X"=w285) -> ("slope"=w282:dbl, "intercept"=w283:dbl)  [unwired: 9 in, 3 out]
    n157 = call <vilib>:"Correlation Coefficient.vi"("Y"=w280, "X"=w285) -> ("correlation coefficient r"=w274:dbl)  [unwired: 8 in, 1 out]
    n158 = Multiply(x="bkank position", y=w282) -> (x*y=w284:dbl)
    n159 = Square(x=w274) -> (x^2=→"R^2":dbl)
    n160 = Add(x=w284, y=w283) -> (x+y=w279:dbl)
    n161 = Power Of 10(x=w279) -> (10^x=→"MESF":dbl)
    "loop index for stat analysis" <- w264
  }
